vi "Configure ARB.vi"(7 "Channel Name":string="0", 8 "error in (no error)":errorcluster, 9 "Amplitude":dbl, 10 "Start Freq.":dbl, 11 "Arb in":refnum<k15>) -> (0 "error out":errorcluster, 3 "Arb out":refnum<k15> caption="Instrument Handle Out")   [LabVIEW 2023, in "Bode Plot - PXI.lvlib"]
doc: "Configures the arbitrary waveform generator and initializes the reference."
uses:
  Bode Plot - PXI.lvlib
  <instrlib>/niFgen/niFgen.llb/niFgen Output Mode.ctl
  <instrlib>/niFgen/niFgen.llb/niFgen Waveform Type.ctl
  <instrlib>/niFgen/niFgen.llb/niFgen Output Impedance.ctl
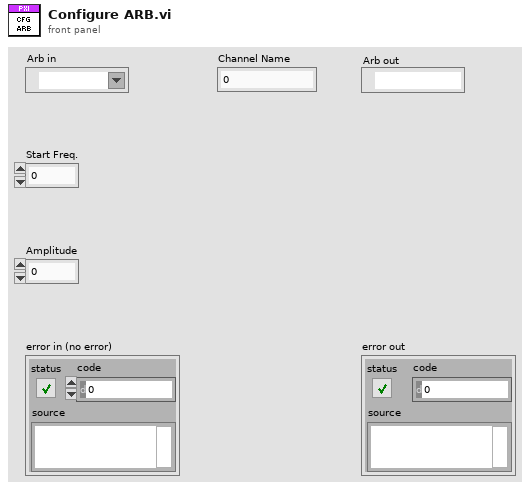
[diagram p1: front panel]
types:
  T1 = typedef "niFgen Output Impedance.ctl" = i32
  T2 = typedef "niFgen Waveform Type.ctl" = i32
  T3 = typedef "niFgen Output Mode.ctl" = u32
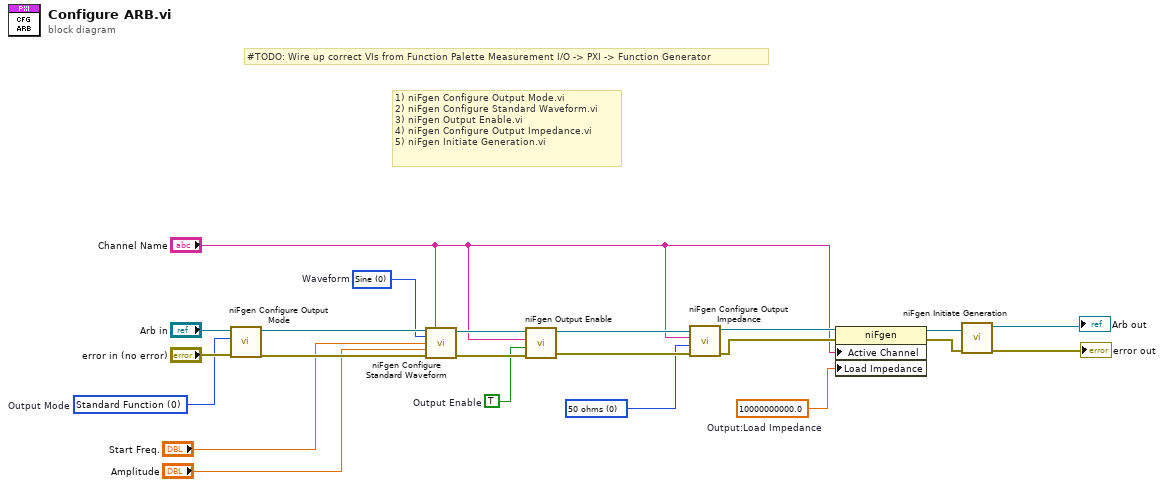
[diagram p0: block diagram]
diagram:
  w6 = 10000000000.0  # Output:Load Impedance
  w9 = T1 0 items=["50 ohms", "75 ohms"] ("Impedance (default: 0=50 ohms)")
  w12 = TRUE  # Output Enable
  w15 = T2 0 items=["Sine", "Square", "Triangle", "Ramp Up", "Ramp Down", "DC", "Noise", "User"]  # Waveform
  w20 = T3 0 items=["Standard Function", "Frequency List", "Arbitrary Waveform", "Arbitrary Sequence", "Script"]  # Output Mode
  # "1) niFgen Configure Output Mode.vi\n2) niFgen Configure Standard Waveform.vi\n3) niFgen Output Enable.vi\n4) niFgen Configure Output Impedance.vi\n5) niFgen Initiate Generation.vi"
  # "#TODO: Wire up correct VIs from Function Palette Measurement I/O -> PXI -> Function Generator"
  n1 = call <instrlib>:"niFgen Configure Output Mode.vi"("error in (no error)"="error in (no error)", "Output Mode (default: 0=Standard Function)"=w20, "Instrument Handle"="Arb in") -> ("error out"=w18:errorcluster, "Instrument Handle Out"=w19:refnum<k15>)  [unwired: 6 in]
  n2 = call <instrlib>:"niFgen Configure Standard Waveform.vi"("Instrument Handle"=w19, "Channel Name"="Channel Name", "Waveform"=w15, "Frequency"="Start Freq.", "Amplitude"="Amplitude", "error in (no error)"=w18) -> ("Instrument Handle Out"=w14:refnum<k15>, "error out"=w13:errorcluster)  [unwired: 8 in]
  n3 = call <instrlib>:"niFgen Output Enable.vi"("error in (no error)"=w13, "Output Enable (default: True)"=w12, "Channel Name"="Channel Name", "Instrument Handle"=w14) -> ("error out"=w10:errorcluster, "Instrument Handle Out"=w11:refnum<k15>)  [unwired: 6 in]
  n4 = call <instrlib>:"niFgen Configure Output Impedance.vi"("error in (no error)"=w10, "Impedance (default: 0=50 ohms)"=w9, "Channel Name"="Channel Name", "Instrument Handle"=w11) -> ("error out"=w7:errorcluster, "Instrument Handle Out"=w8:refnum<k15>)  [unwired: 6 in]
  n5 = property class="niFgen"(reference=w8, error in=w7, "Active Channel"="Channel Name", "Load Impedance"=w6) -> (reference out=w5:refnum<k15>, error out=w4:errorcluster)
  n6 = call <instrlib>:"niFgen Initiate Generation.vi"("error in (no error)"=w4, "Instrument Handle"=w5) -> ("error out"=→"error out":errorcluster, "Instrument Handle Out"=→"Arb out":refnum<k15>)  [unwired: 8 in]
